vi "Set Attachments2.vi"(0 "handles cluster in":T1 caption="ハンドルクラスター入力", 5 "attachments":path[](array[path]) caption="添付", 11 "error in (no error)":errorcluster caption="エラー入力（エラーなし）") -> (4 "handles cluster out":T1 caption="ハンドルクラスター出力", 15 "error out":errorcluster caption="エラー出力")   [LabVIEW 2015]
doc: "Eメールに含めるファイルのリストを設定します。実行前に添付に指定された値は上書きされます。"
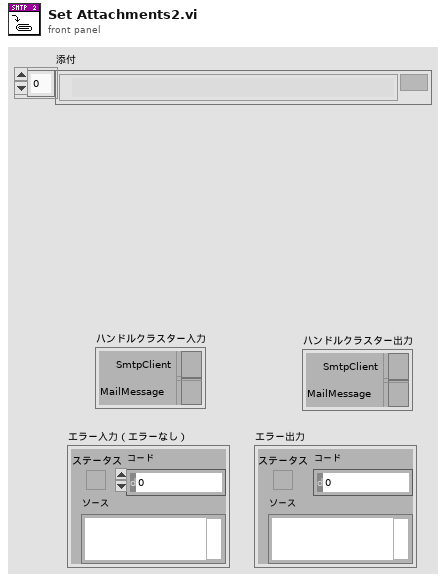
[diagram p1: front panel]
types:
  T1 = cluster{"SmtpClient":refnum<k24>, "MailMessage":refnum<k24>}
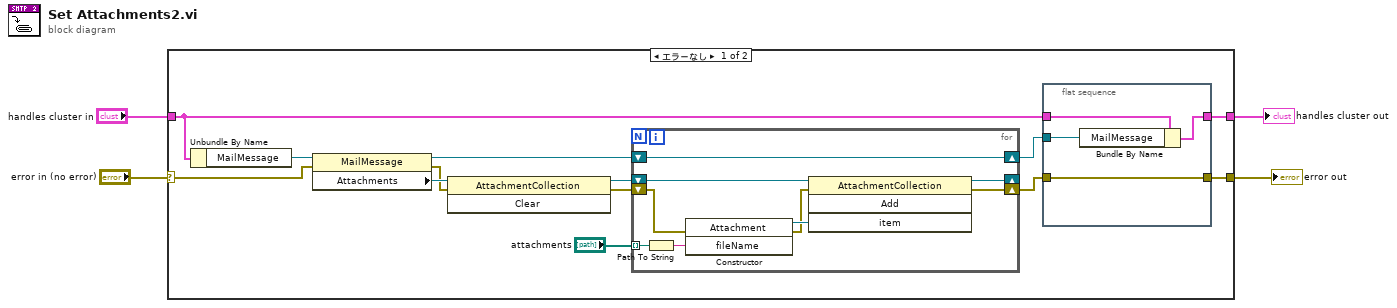
[diagram p0: block diagram]
diagram:
  n1 = case shown="エラーなし" "error in (no error)" {
    selector: "error in (no error)" -> [w12 w32]
    tunnel: [w10 w32] -> w3
    tunnel: "handles cluster in" -> [w17 w31]
    tunnel: [w16 w31] -> w1
    frame No Error {
      n2 = Unbundle By Name(w17) -> ("MailMessage"=w14:refnum<k24>)
      n3 = property class="MailMessage"(reference=w14, error in=w12) -> (reference out=w15:refnum<k24>, error out=w7:errorcluster, "Attachments"=w8:refnum<k24>)
      n4 = invoke class="AttachmentCollection" method="Clear"(reference=w8, error in=w7) -> (reference out=w6:refnum<k24>, error out=w5:errorcluster)  [unwired: 1 in, 1 out]
      n5 = for {
        shift-right: [w19] -> _
        shift-left: w6 -> [w26]
        shift-right: [w20] -> w9
        shift-left: w5 -> [w22]
        shift-right: [w18] -> w11
        shift-left: w15 -> [w18]
        tunnel: "attachments" -> [w23] mode=indexing
        n6 = Path To String(path=w23) -> (string=w25:string)
        n7 = constructor class="Attachment"(error in=w22, "fileName"=w25) -> (reference out=w24:refnum<k24>, error out=w21:errorcluster)  [unwired: 2 in, 2 out]
        n8 = invoke class="AttachmentCollection" method="Add"(reference=w26, error in=w21, "item"=w24) -> (reference out=w19:refnum<k24>, error out=w20:errorcluster)  [unwired: 1 in, 2 out]
      }
      n9 = flat-sequence {
        tunnel: w17 -> [w30]
        tunnel: [w29] -> w16
        tunnel: w11 -> [w28]
        tunnel: [w27] -> w10
        tunnel: w9 -> [w27]
        frame #0 {
          n10 = Bundle By Name(cluster=w30, "MailMessage"=w28) -> (w29:T1)
        }
      }
    }
    frame Error {
    }
  }
  "handles cluster out" <- w1
  "error out" <- w3
